vi "STM上位机-Client.vi"() -> ()   [LabVIEW 2015]
uses:
  <vilib>/Math Plots/3D Math Plots/3D Surface/3D Surface XCtrl/3D Surface.xctl
  <vilib>/NI/STM/TCP/TCP Read Options.ctl
  <vilib>/vision/Image Controls.llb/IMAQ Image.ctl
  <vilib>/Analysis/6fits.llb/Curve Fitting Criteria.ctl
  <vilib>/NI/STM/TCP/Read Meta Data (TCP Ref).vi
  <vilib>/NI/STM/TCP/Get Connection Reference (TCP).vi
  <vilib>/NI/STM/TCP/Read Meta Data (TCP Clst).vi
  <vilib>/NI/STM/TCP/Write Message (TCP).vi
  <vilib>/NI/STM/TCP/Read Message (TCP).vi
  <vilib>/Math Plots/3D Math Plots/3D Surface/3D Surface Datatype/Public/Plot Helper (Vector).vi
  <vilib>/NI/STM/NI STM.lvlib
  <vilib>/Math Plots/3D Math Plots/3D Surface/3D Surface Datatype/3D Surface Datatype.lvclass
  <vilib>/Analysis/NI_AALPro.lvlib
panel:
  in  "树形":string(tree)
  in  "Tab Control 3":T1(tab)
  in  "实验人员":string
  in  "实验地点":string
  in  "激光波长":dbl
  in  "自动前进":bool
  in  "自动后退":bool
  in  "中心点":u16(ring) items=["自动", "自动获取质心", "手动取心"]
  in  "步进距离":u16(ring) items=["1mm", "2mm", "4mm", "8mm"]
  in  "触发":bool
  in  "记录数据":bool
  in  "删除数据":bool
  in  "计算M2因子":bool
  in  "是否加中心线":bool
  in  "是否加椭圆线":bool
  out "周长(mm)":dbl
  out "质心坐标X":dbl
  out "质心坐标Y":dbl
  out "面积(mm2)":dbl
  in  "保存数据":bool
  in  "保存边缘检测图像":bool
  in  "保存3D图像":bool
  in  "保存伪彩色图像":bool
  out "位置              长轴半径         短轴半径":string[][](array[string])
  in  "Tab Control 2":T2(tab)
  out "长轴原曲线":dbl[](graph)
  out "长轴拟合曲线":dbl[](graph)
  out "长轴长度":dbl
  out "短轴M2因子":dbl
  out "长轴M2因子":dbl
  out "长轴束腰位置Z0":dbl
  out "长轴束腰直径":dbl
  out "长轴瑞利长度":dbl
  out "长轴光束发散角":dbl
  out "短轴束腰位置Z0":dbl
  out "短轴束腰直径":dbl
  out "短轴瑞利长度":dbl
  out "短轴光束发散角":dbl
  out "手动取点x":i32
  out "是否手动取点":bool
  out "短轴长度":dbl
  out "位置":dbl
  out "3D":u8[](array[numeric])
  out "短轴半径um":dbl
  out "长轴半径um":dbl
  out "短轴原曲线":dbl[](graph)
  out "短轴拟合曲线":dbl[](graph)
  out "纵轴原曲线":dbl[](graph)
  out "纵轴拟合曲线":dbl[](graph)
  out "横轴原曲线":dbl[](graph)
  out "横轴拟合曲线":dbl[](graph)
  in  "Tab Control":enum32{"边缘检测", "3D图像", "伪彩色图像", "三维成像"}(tab)
  out "边缘检测":T3(plugin-control)
  out "3D图像":T3(plugin-control)
  out "伪彩色图像":T3(plugin-control)
  out "三维图像":refnum<class "3D Plot Datatype.lvclass">[](xcontrol) caption="3D Surface"
  in  "读取3D数据":bool
  in  "关闭程序":bool
  out "手动取点y":i32
  # "长轴原曲线"
  # "长轴拟合曲线"
  # "短轴原曲线"
  # "短轴拟合曲线"
  # "纵轴原曲线"
  # "纵轴拟合曲线"
  # "横轴原曲线"
  # "横轴拟合曲线"
  # "三维成像"
  # "-10.00\n\n\n\n-5.00\n\n\n\n-0.00"
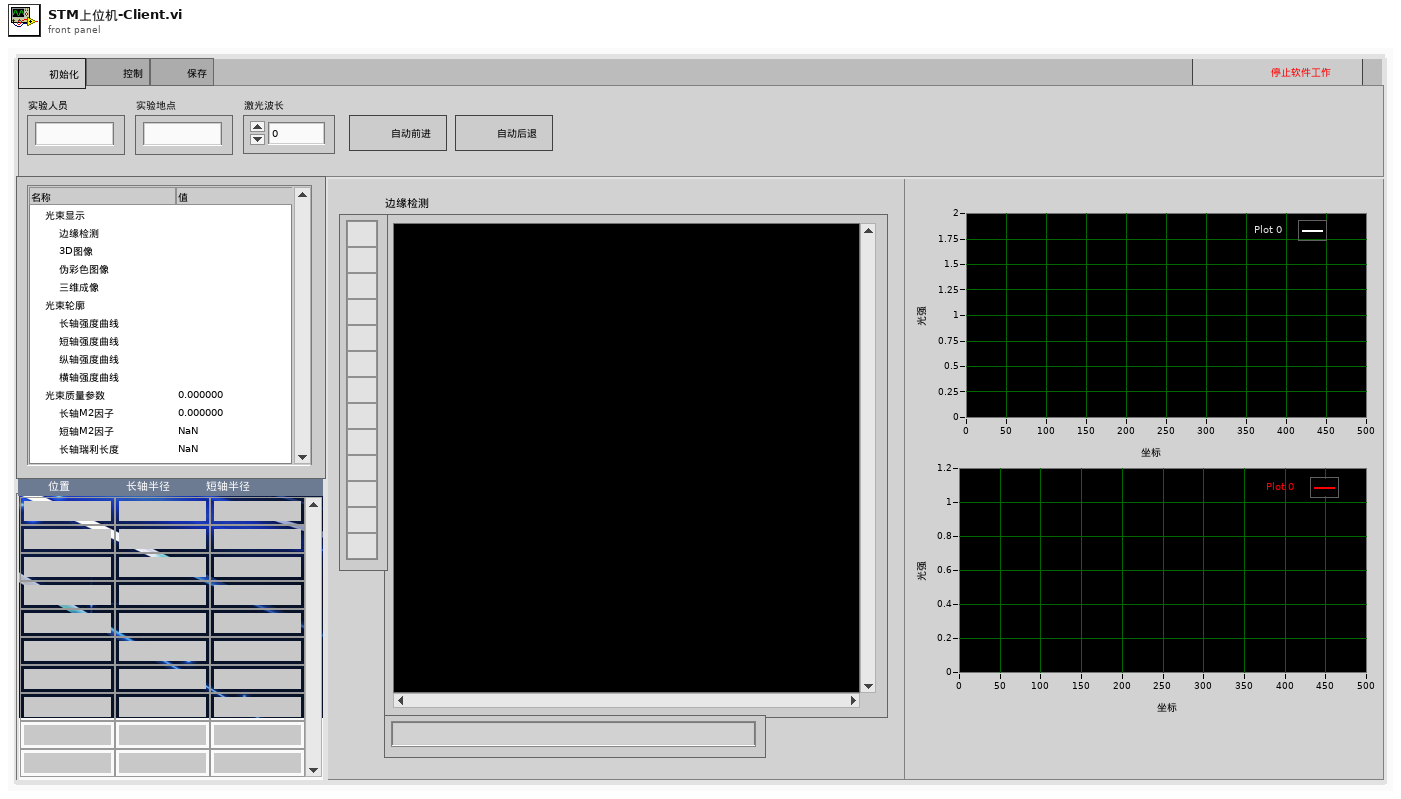
[diagram p1: front panel]
types:
  T1 = enum32{"        初始化", "          控制", "          保存"}
  T2 = enum32{"长轴原曲线", "长轴拟合曲线 ", "短轴原曲线", "短轴拟合曲线", "纵轴原曲线  ", "纵轴拟合曲线  ", "横轴原曲线 ", "横轴拟合曲线 "}
  T3 = typedef "IMAQ Image.ctl" = refnum<image>
  T4 = typedef "NI STM.lvlib/TCP Connection Info.ctl" = cluster{"connection ID":refnum<k5>, "meta data":T5[]}
  T5 = typedef "NI STM.lvlib/MetaDataElement.ctl" = string
  T6 = typedef "NI_AALPro.lvlib/Curve Fitting Criteria.ctl" = u16
  T7 = typedef "NI STM.lvlib/TCP Read Options.ctl" = cluster{"ignore timeout error":bool, "timeout ms (1000)":i32}
  T8 = cluster{"周长":dbl, "面积":dbl, "3D":u8[], "灰度图像":T3, "3D view":T3, "滤波":T3, "边缘检测":T3, "3D图像":T3, "质心坐标X":sgl, "质心坐标Y":sgl, "第一点y值，x=0":dbl, "第二点y值，x=639":dbl, "第一点x值，y=0":dbl, "第二点x值，y=479":dbl, "短轴半径um":dbl, "长轴半径um":dbl, "长轴长度":dbl, "短轴长度":dbl, "短轴原曲线":dbl[], "长轴拟合":dbl[], "纵轴拟合":dbl[], "横轴拟合":dbl[], "长轴原曲线":dbl[], "纵轴原曲线":dbl[], "横轴原曲线":dbl[], "短轴拟合":dbl[], "位置":dbl}
  T9 = cluster{"Global Rectangle":i32[], "Contours":cluster{"Contour Type":u32, "ROI Type":u32, "Points":i32[]}[]}
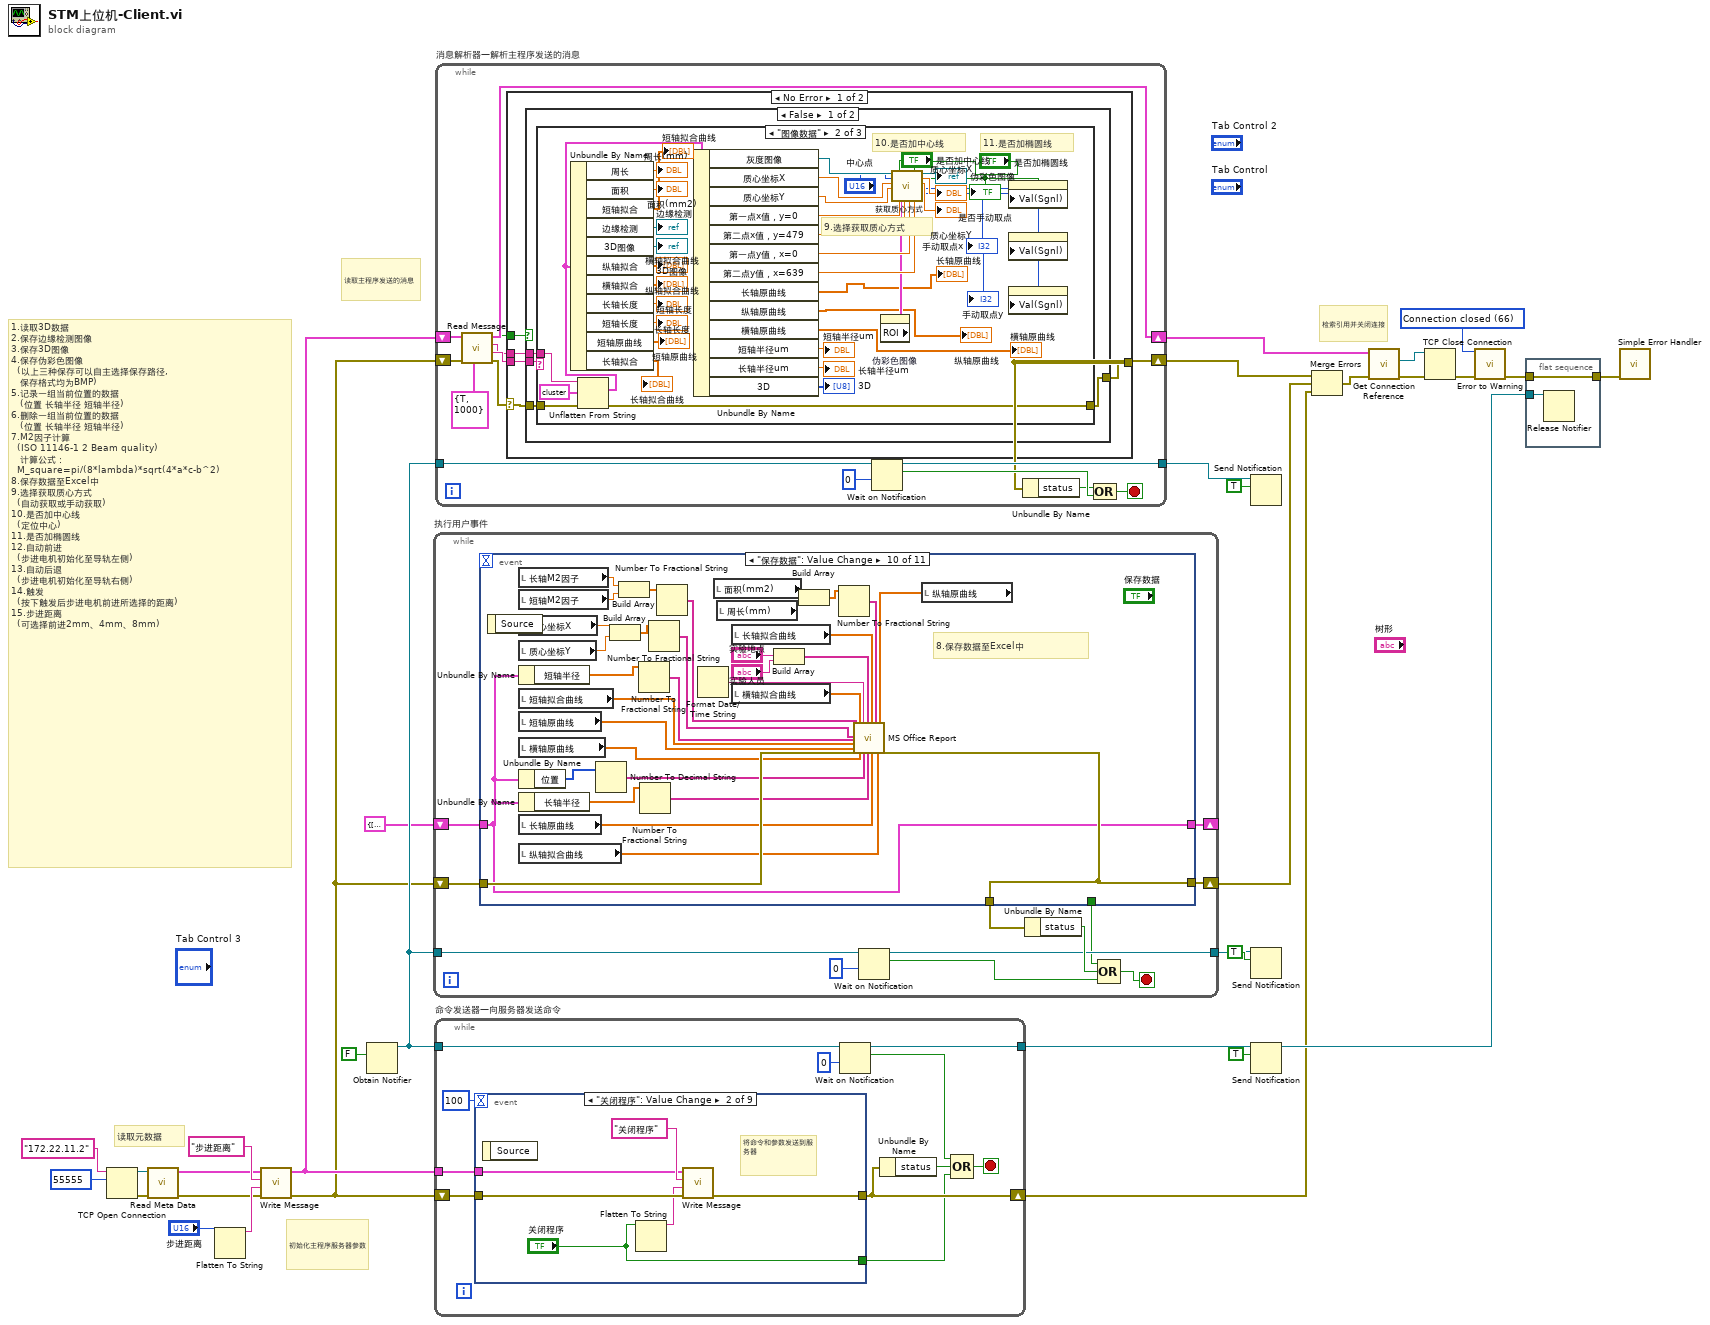
[diagram p0: block diagram]
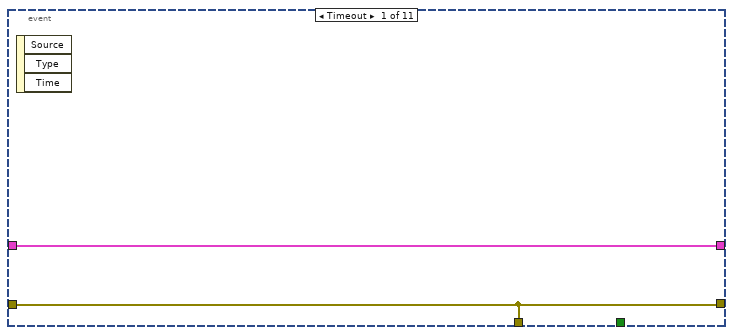
[diagram p2: hidden frame]
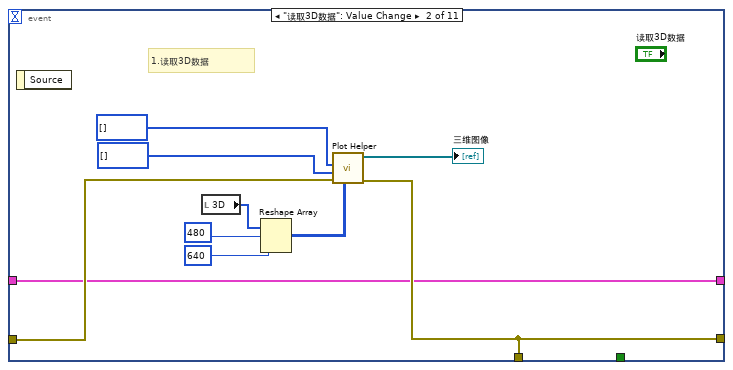
[diagram p3: hidden frame]
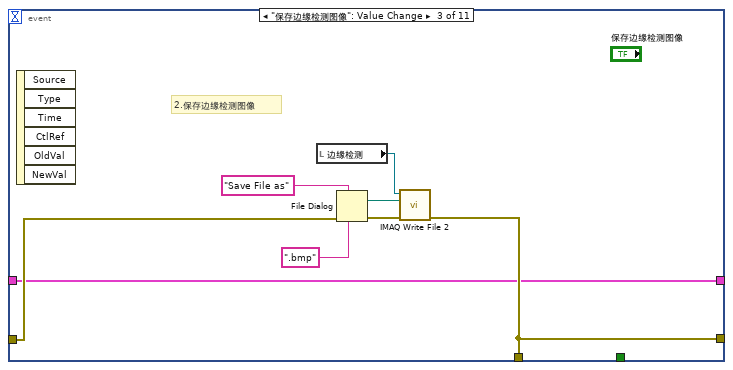
[diagram p4: hidden frame]
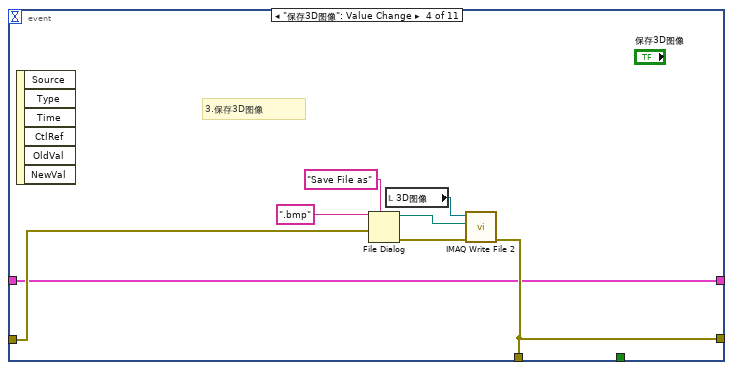
[diagram p5: hidden frame]
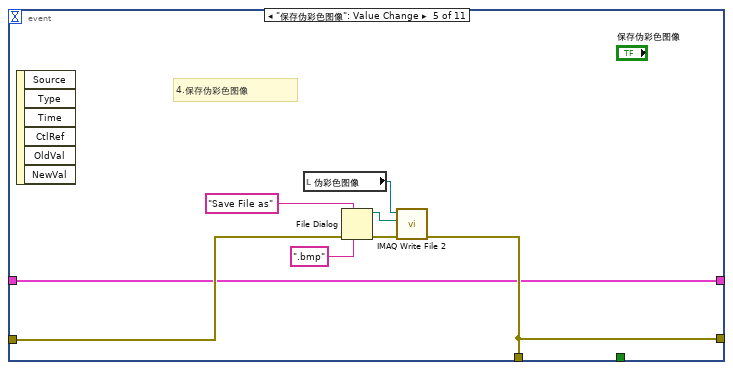
[diagram p6: hidden frame]
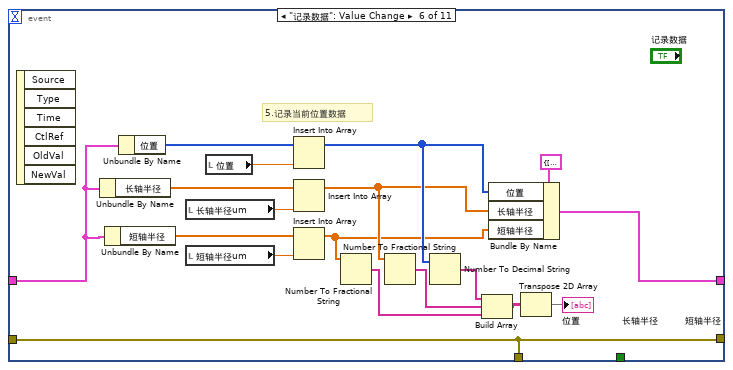
[diagram p7: hidden frame]
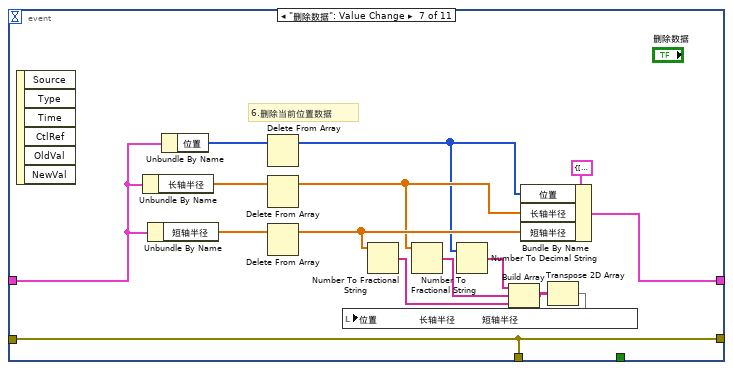
[diagram p8: hidden frame]
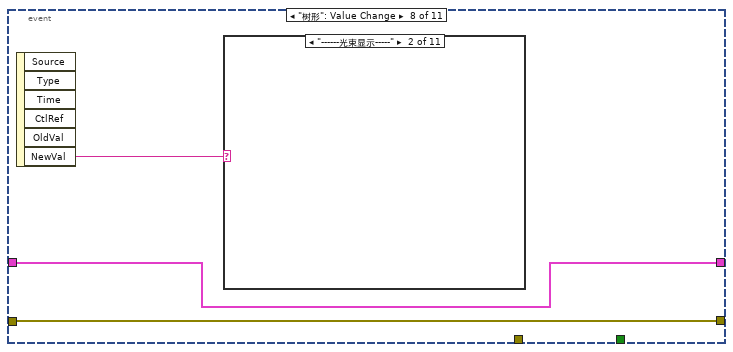
[diagram p9: hidden frame]
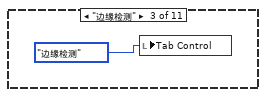
[diagram p11: hidden frame]
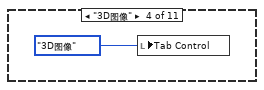
[diagram p12: hidden frame]
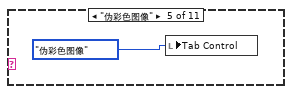
[diagram p13: hidden frame]
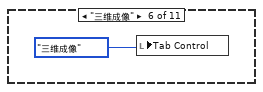
[diagram p14: hidden frame]
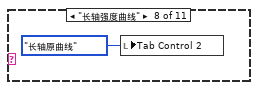
[diagram p16: hidden frame]
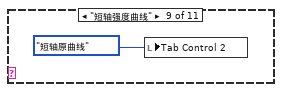
[diagram p17: hidden frame]
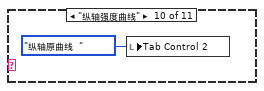
[diagram p18: hidden frame]
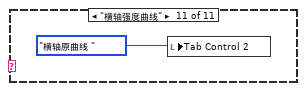
[diagram p19: hidden frame]
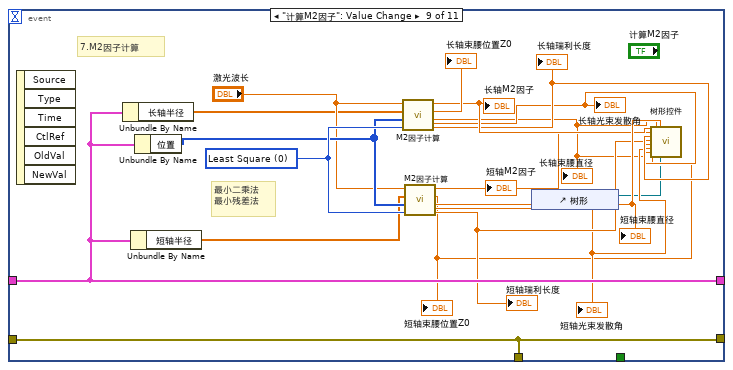
[diagram p20: hidden frame]
diagram:
  w28 = 66 items=["No Error", "Argument Error", "Memory Full", "Out of Zone", "End of File", "File Already Open", "Generic File IO Error", "File Not Found", "File Permission Error", "Disk Full", "Duplicate Path", "Too Many Files Open", "Not Enabled", "Resource File Not Found", "Cannot Add Resource", "Resource Not Found", "Image Not Found", "Image Memory Error", "Pen Does Not Exist", "Config Bad Type", "Config Token Not Found", "Config Parse Error", "Config Memory Error", "Bad External Code Format", "Bad External Code Offset", "External Code Not Present", "Null Window", "Destroy Window Mixup", "Null Menu", "Print Aborted", "Bad Print Record", "Print Driver Error", "Windows Error During Print", "Memory Error During Print", "Print Dialog Error", "Generic Print Error", "Invalid Device Refnum", "Device Not Found", "Device Parameter Error", "Device Unit Error", "Can't Open Device", "Device Call Aborted", "Generic Error", "Cancelled By User", "Object ID Too Low", "Object ID Too High", "Object Not In Heap", "Unknown Heap", "Bad DefProc ID", "DefProc Not In Table", "Message Out Of Range", "Null Method", "Unknown Message", "Manager Call Not Supported", "Bad address", "Connection In progress", "Connection timed out", "Connection is already in progress", "Network attribute not supported", "Network error", "Address in use", "System out of memory", "Connection aborted", "Connection refused", "Connection is not connected", "Connection is already connected", "Connection closed", "Initialize error (interapplication manager)", "Bad occurrence", "Wait on unbound occurrence handler", "Occurrence queue overflow", "Bad path", "Semaphore not signaled", "Unrecognized type (interapplication manager)"] ("1st Error to Convert")
  # "检索引用并关闭连接"
  # "读取元数据"
  # "读取主程序发送的消息"
  # "初始化主程序服务器参数"
  # "1.读取3D数据\n2.保存边缘检测图像\n3.保存3D图像\n4.保存伪彩色图像\n  (以上三种保存可以自主选择保存路径,   \n   保存格式均为BMP)\n5.记录一组当前位置的数据\n   (位置 长轴半径 短轴半径)\n6.删除一组当前位置的数据\n   (位置 长轴半径 短轴半径)\n7.M2因子计算\n  (ISO 11146-1 2 Beam quality)\n   计算公式：\n  M_square=pi/(8*lambda)*sqrt(4*a*c-b^2)\n8.保存数据至Excel中\n9.选择获取质心方式\n  (自动获取或手动获取)\n10.是否加中心线\n  (定位中心)\n11.是否加椭圆线\n12.自动前进\n  (步进电机初始化至导轨左侧)\n13.自动后退\n  (步进电机初始化至导轨右侧)\n14.触发\n  (按下触发后步进电机前进所选择的距离)\n15.步进距离\n  (可选择前进2mm、4mm、8mm)"
  n1 = TCP Open Connection(address="172.22.11.2" ("Target IP Address"), remote port or service name=u16 55555 ("remote port")) -> (connection ID=w32:refnum<k5>, error out=w31:errorcluster)  [unwired: 1 in, 2 out]
  n2 = call-poly "Read Meta Data.vi"("error in"=w31, "connection ID"=w32) -> ("error out"=w3:errorcluster, "connection info out"=w5:T4)  [unwired: 1 in, 7 out]
  n3 = Flatten To String(anything="步进距离") -> (data string=w7:string)  [unwired: 2 in, 3 out]
  n4 = call-poly "Write Message.vi"("error in"=w3, "data"=w7, "name"="步进距离" ("Name"), "connection info in"=w5) -> ("error out"=w2:errorcluster, "connection info out"=w4:T4)  [unwired: 1 in, 5 out]
  n5 = Obtain Notifier(notification data type=FALSE) -> (notifier out=w12:refnum<notifier>)  [unwired: 3 in, 2 out]
  n6 = while "执行用户事件" {
    shift-right: [w36] -> w9
    shift-left: w2 -> [w37]
    tunnel: w12 -> [w42]
    tunnel: [w40] -> w10
    shift-right: [w33] -> _
    shift-left: cluster{"位置":i32[], "长轴半径":dbl[], "短轴半径":dbl[]} {"位置"=[], "长轴半径"=[], "短轴半径"=[]} -> [w38]
    stop <- w39 stop-if-true
    n7 = event shown="[9] \"保存数据\": Value Change" {
      selector: _ -> [_ _ _ _ _ _ _ _ _ _ _]
      dyn-events: _ -> [_ _ _ _ _ _ _ _ _ _ _]
      timeout: _ -> [_ _ _ _ _ _ _ _ _ _ _]
      tunnel: w38 -> [w46 w48 w57 w65 w73 w95 w112 w115 w139 w148 _]
      tunnel: w37 -> [w45 w51 w59 w67 w76 w89 w107 w114 w138 w154 _]
      tunnel: [w45 w49 w58 w66 w75 w89 w107 w114 w138 w153 _] -> w36
      tunnel: [w45 w49 w58 w66 w75 w89 w107 _ w138 w153 _] -> w35
      tunnel: [_ _ _ _ _ _ _ _ _ _ TRUE] -> w34
      tunnel: [w46 w48 w57 w65 w73 w90 w108 w115 w139 w148 _] -> w33
      event Timeout {
        n8 = event-data() -> ()  [unwired: 1 in, 3 out]
      }
      event "读取3D数据": Value Change {
        # "1.读取3D数据"
        n9 = event-data() -> ()  [unwired: 1 in, 1 out]
        n10 = local read "3D"() -> (w50:u8[])
        n11 = Reshape Array(w50, 480 ("dimension size"), 640 ("dimension size")) -> (w54:u8[][])
        n12 = call-poly <vilib>:"Plot Helper.vi"("z matrix"=w54, "error in (no error)"=w51, "y vector"=i32[] [] ("3D"), "x vector"=i32[] [] ("3D")) -> ("error out"=w49:errorcluster, "3D Plot lvclass Array out"=→"三维图像":refnum<class "3D Plot Datatype.lvclass">[])  [unwired: 2 in, 4 out]
      }
      event "保存边缘检测图像": Value Change {
        # "2.保存边缘检测图像"
        n13 = event-data() -> ()  [unwired: 1 in, 6 out]
        n14 = local read "边缘检测"() -> (w60:T3)
        n15 = File Dialog(6:".bmp" ("pattern (all files)"), 7:"Save File as" ("prompt"), 8:w59) -> (0:w61:errorcluster, 3:w64:path)  [unwired: 4 in, 2 out]
        n16 = call-poly "IMAQ Write File 2"("error in (no error)"=w61, "File Path"=w64, "Image"=w60) -> ("error out"=w58:errorcluster)  [unwired: 7 in, 1 out]
      }
      event "保存3D图像": Value Change {
        # "3.保存3D图像"
        n17 = event-data() -> ()  [unwired: 1 in, 6 out]
        n18 = File Dialog(6:".bmp" ("pattern (all files)"), 7:"Save File as" ("prompt"), 8:w67) -> (0:w69:errorcluster, 3:w72:path)  [unwired: 4 in, 2 out]
        n19 = local read "3D图像"() -> (w68:T3)
        n20 = call-poly "IMAQ Write File 2"("error in (no error)"=w69, "File Path"=w72, "Image"=w68) -> ("error out"=w66:errorcluster)  [unwired: 7 in, 1 out]
      }
      event "保存伪彩色图像": Value Change {
        # "4.保存伪彩色图像"
        n21 = event-data() -> ()  [unwired: 1 in, 6 out]
        n22 = local read "伪彩色图像"() -> (w74:T3)
        n23 = File Dialog(6:".bmp" ("pattern (all files)"), 7:"Save File as" ("prompt"), 8:w76) -> (0:w77:errorcluster, 3:w80:path)  [unwired: 4 in, 2 out]
        n24 = call-poly "IMAQ Write File 2"("error in (no error)"=w77, "File Path"=w80, "Image"=w74) -> ("error out"=w75:errorcluster)  [unwired: 7 in, 1 out]
      }
      event "记录数据": Value Change {
        # "5.记录当前位置数据"
        n25 = event-data() -> ()  [unwired: 1 in, 6 out]
        n26 = Unbundle By Name(w95) -> ("长轴半径"=w97:dbl[])
        n27 = Unbundle By Name(w95) -> ("短轴半径"=w98:dbl[])
        n28 = Unbundle By Name(w95) -> ("位置"=w96:i32[])
        n29 = local read "长轴半径um"() -> (w93:dbl)
        n30 = local read "短轴半径um"() -> (w92:dbl)
        n31 = local read "位置"() -> (w94:dbl)
        n32 = Insert Into Array(array=w96, new element=w94) -> (w88:i32[])  [unwired: 1 in]
        n33 = Insert Into Array(array=w97, new element=w93) -> (w87:dbl[])  [unwired: 1 in]
        n34 = Insert Into Array(array=w98, new element=w92) -> (w86:dbl[])  [unwired: 1 in]
        n35 = Number To Fractional String(number=w86) -> (F-format string=w83:string[])  [unwired: 3 in]
        n36 = Number To Fractional String(number=w87) -> (F-format string=w82:string[])  [unwired: 3 in]
        n37 = Number To Decimal String(number=w88) -> (decimal integer string=w81:string[])  [unwired: 1 in]
        n38 = Build Array(w81, w82, w83) -> (w85:string[][])
        n39 = Bundle By Name(cluster=cluster{"位置":i32[], "长轴半径":dbl[], "短轴半径":dbl[]} {"位置"=[], "长轴半径"=[], "短轴半径"=[]}, "位置"=w88, "长轴半径"=w87, "短轴半径"=w86) -> (w90:cluster{"位置":i32[], "长轴半径":dbl[], "短轴半径":dbl[]})
        n40 = Transpose 2D Array(2D array=w85) -> (transposed array=→"位置              长轴半径         短轴半径":string[][])
      }
      event "删除数据": Value Change {
        # "6.删除当前位置数据"
        n41 = event-data() -> ()  [unwired: 1 in, 6 out]
        n42 = Unbundle By Name(w112) -> ("长轴半径"=w110:dbl[])
        n43 = Unbundle By Name(w112) -> ("短轴半径"=w109:dbl[])
        n44 = Unbundle By Name(w112) -> ("位置"=w111:i32[])
        n45 = Delete From Array(array=w111) -> (array with subset deleted=w100:i32[])  [unwired: 2 in, 1 out]
        n46 = Delete From Array(array=w110) -> (array with subset deleted=w101:dbl[])  [unwired: 2 in, 1 out]
        n47 = Delete From Array(array=w109) -> (array with subset deleted=w102:dbl[])  [unwired: 2 in, 1 out]
        n48 = Number To Fractional String(number=w102) -> (F-format string=w105:string[])  [unwired: 3 in]
        n49 = Number To Fractional String(number=w101) -> (F-format string=w104:string[])  [unwired: 3 in]
        n50 = Number To Decimal String(number=w100) -> (decimal integer string=w103:string[])  [unwired: 1 in]
        n51 = Build Array(w103, w104, w105) -> (w106:string[][])
        n52 = Bundle By Name(cluster=cluster{"位置":i32[], "长轴半径":dbl[], "短轴半径":dbl[]} {"位置"=[], "长轴半径"=[], "短轴半径"=[]}, "位置"=w100, "长轴半径"=w101, "短轴半径"=w102) -> (w108:cluster{"位置":i32[], "长轴半径":dbl[], "短轴半径":dbl[]})
        n53 = Transpose 2D Array(2D array=w106) -> (transposed array=w99:string[][])
        n54 = local write "位置              长轴半径         短轴半径"(w99) -> ()
      }
      event "树形": Value Change {
        n55 = event-data() -> ("NewVal"=w116:string)  [unwired: 1 in, 5 out]
        n56 = case shown="\"------光束显示-----\"" w116 {
          frame "假", Default {
          }
          frame "------光束显示-----" {
          }
          frame "边缘检测" {
            n57 = local write "Tab Control"(enum32{"边缘检测", "3D图像", "伪彩色图像", "三维成像"}."边缘检测" ("Tab Control")) -> ()
          }
          frame "3D图像" {
            n58 = local write "Tab Control"(enum32{"边缘检测", "3D图像", "伪彩色图像", "三维成像"}."3D图像" ("Tab Control")) -> ()
          }
          frame "伪彩色图像" {
            n59 = local write "Tab Control"(enum32{"边缘检测", "3D图像", "伪彩色图像", "三维成像"}."伪彩色图像" ("Tab Control")) -> ()
          }
          frame "三维成像" {
            n60 = local write "Tab Control"(enum32{"边缘检测", "3D图像", "伪彩色图像", "三维成像"}."三维成像" ("Tab Control")) -> ()
          }
          frame "------光束轮廓-----" {
          }
          frame "长轴强度曲线" {
            n61 = local write "Tab Control 2"(T2."长轴原曲线" ("Tab Control 2")) -> ()
          }
          frame "短轴强度曲线" {
            n62 = local write "Tab Control 2"(T2."短轴原曲线" ("Tab Control 2")) -> ()
          }
          frame "纵轴强度曲线" {
            n63 = local write "Tab Control 2"(T2."纵轴原曲线  " ("Tab Control 2")) -> ()
          }
          frame "横轴强度曲线" {
            n64 = local write "Tab Control 2"(T2."横轴原曲线 " ("Tab Control 2")) -> ()
          }
        }
      }
      event "计算M2因子": Value Change {
        w142 = T6 0 items=["Least Square", "Least Absolute Residual", "Bisquare"] ("method")
        # "7.M2因子计算"
        # "最小二乘法\n最小残差法"
        n65 = event-data() -> ()  [unwired: 1 in, 6 out]
        n66 = Unbundle By Name(w139) -> ("长轴半径"=w136:dbl[])
        n67 = Unbundle By Name(w139) -> ("短轴半径"=w137:dbl[])
        n68 = Unbundle By Name(w139) -> ("位置"=w141:i32[])
        n69 = call "M2因子计算.vi"("method"=w142, "位置"=w141, "光斑半径"=w136, "激光波长"="激光波长") -> ("瑞利长度"=w131:dbl, "束腰直径"=w127:dbl, "束腰位置Z0"=→"长轴束腰位置Z0":dbl, "M2因子"=w133:dbl, "光束发散角"=w129:dbl)  [unwired: 3 in]
        "长轴M2因子" <- w133
        "长轴束腰直径" <- w127
        "长轴瑞利长度" <- w131
        "长轴光束发散角" <- w129
        n70 = call "M2因子计算.vi"("method"=w142, "位置"=w141, "光斑半径"=w137, "激光波长"="激光波长") -> ("瑞利长度"=w130:dbl, "束腰直径"=w134:dbl, "束腰位置Z0"=w126:dbl, "M2因子"=w132:dbl, "光束发散角"=w128:dbl)  [unwired: 3 in]
        "短轴M2因子" <- w132
        "短轴束腰位置Z0" <- w126
        "短轴束腰直径" <- w134
        "短轴瑞利长度" <- w130
        "短轴光束发散角" <- w128
        n71 = control-ref of="树形"() -> (w125:refnum<vi>)
        n72 = call "树形控件.vi"("长轴M2因子"=w133, "短轴M2因子"=w132, "长轴瑞利长度"=w131, "短轴瑞利长度"=w130, "长轴光束发散角"=w129, "短轴光束发散角"=w128, "长轴束腰位置Z0"=w127, "短轴束腰位置Z0"=w126, "长轴束腰直径"=w127, "短轴束腰直径"=w134, "Tree引用句柄"=w125) -> ()  [unwired: 17 in]
      }
      event "保存数据": Value Change {
        # "8.保存数据至Excel中"
        n73 = event-data() -> ()  [unwired: 1 in, 1 out]
        n74 = local read "长轴M2因子"() -> (w163:dbl)
        n75 = local read "短轴M2因子"() -> (w162:dbl)
        n76 = local read "质心坐标X"() -> (w159:dbl)
        n77 = local read "质心坐标Y"() -> (w158:dbl)
        n78 = Unbundle By Name(w148) -> ("短轴半径"=w151:dbl[])
        n79 = local read "短轴拟合曲线"() -> (w156:dbl[])
        n80 = local read "短轴原曲线"() -> (w155:dbl[])
        n81 = local read "横轴原曲线"() -> (w152:dbl[])
        n82 = Unbundle By Name(w148) -> ("位置"=w147:i32[])
        n83 = Unbundle By Name(w148) -> ("长轴半径"=w146:dbl[])
        n84 = local read "长轴原曲线"() -> (w150:dbl[])
        n85 = local read "纵轴拟合曲线"() -> (w149:dbl[])
        n86 = Number To Decimal String(number=w147) -> (decimal integer string=w145:string[])  [unwired: 1 in]
        n87 = Build Array(w159, w158) -> (w160:dbl[])
        n88 = Build Array(w163, w162) -> (w164:dbl[])
        n89 = Number To Fractional String(number=w151) -> (F-format string=w143:string[])  [unwired: 3 in]
        n90 = Number To Fractional String(number=w146) -> (F-format string=w144:string[])  [unwired: 3 in]
        n91 = Number To Fractional String(number=w160) -> (F-format string=w157:string[])  [unwired: 3 in]
        n92 = Number To Fractional String(number=w164) -> (F-format string=w161:string[])  [unwired: 3 in]
        n93 = Format Date/Time String() -> (date/time string=w166:string)  [unwired: 3 in]
        n94 = local read "面积(mm2)"() -> (w174:dbl)
        n95 = local read "周长(mm)"() -> (w173:dbl)
        n96 = local read "长轴拟合曲线"() -> (w170:dbl[])
        n97 = local read "横轴拟合曲线"() -> (w165:dbl[])
        n98 = Build Array("实验人员", "实验地点") -> (w167:string[])
        n99 = Build Array(w174, w173) -> (w172:dbl[])
        n100 = Number To Fractional String(number=w172) -> (F-format string=w171:string[])  [unwired: 3 in]
        n101 = local read "纵轴原曲线"() -> (w175:dbl[])
        n102 = call "MS Office Report"("M2因子"=w161, "XY"=w157, "短轴半径"=w143, "短轴拟合曲线"=w156, "短轴原曲线"=w155, "error in (no error)"=w154, "横轴拟合曲线"=w165, "横轴原曲线"=w152, "时间"=w166, "位置"=w145, "信息"=w167, "长轴半径"=w144, "长轴拟合曲线"=w170, "长轴原曲线"=w150, "周长与面积"=w171, "纵轴拟合曲线"=w149, "纵轴原曲线"=w175) -> ("error out"=w153:errorcluster)  [unwired: 10 in]
      }
      event "关闭程序": Value Change {
        n103 = event-data() -> ()  [unwired: 1 in, 6 out]
      }
    }
    n104 = Wait on Notification(notifier=w42, timeout in ms (-1)=0) -> (notifier out=w40:refnum<notifier>, notification=w41:bool)  [unwired: 2 in, 2 out]
    n105 = Unbundle By Name(w35) -> ("status"=w44:bool)
    n106 = Compound Arithmetic op=OR(w34, w44, w41) -> (w39:bool)
  }
  n107 = while "命令发送器—向服务器发送命令" {
    tunnel: w4 -> [w187]
    shift-right: [w182] -> w13
    shift-left: w2 -> [w186]
    tunnel: w12 -> [w183]
    tunnel: [w177] -> w17
    stop <- w179 stop-if-true
    n108 = event shown="[1] \"关闭程序\": Value Change" {
      selector: _ -> [_ _ _ _ _ _ _ _ _]
      dyn-events: _ -> [_ _ _ _ _ _ _ _ _]
      timeout: 100 -> [_ _ _ _ _ _ _ _ _]
      tunnel: w187 -> [_ w193 w198 w204 w210 w214 w222 w228 w234]
      tunnel: w186 -> [w188 w192 w197 w203 w209 w215 w221 w227 w233]
      tunnel: [_ "关闭程序" _ _ _ _ _ _ _] -> w180
      tunnel: [w188 w190 w196 w202 w208 w216 w220 w226 w232] -> w182
      event Timeout {
        n109 = event-data() -> ()  [unwired: 2 out]
      }
      event "关闭程序": Value Change {
        # "将命令和参数发送到服务器"
        n110 = event-data() -> ()  [unwired: 2 out]
        n111 = Flatten To String(anything="关闭程序") -> (data string=w191:string)  [unwired: 2 in, 3 out]
        n112 = call-poly "Write Message.vi"("error in"=w192, "data"=w191, "name"="关闭程序" ("Name"), "connection info in"=w193) -> ("error out"=w190:errorcluster)  [unwired: 1 in, 6 out]
      }
      event "自动前进": Value Change {
        # "将命令和参数发送到服务器"
        # "12.自动前进"
        n113 = event-data() -> ()  [unwired: 2 out]
        n114 = Flatten To String(anything="自动前进") -> (data string=w199:string)  [unwired: 2 in, 3 out]
        n115 = call-poly "Write Message.vi"("error in"=w197, "data"=w199, "name"="自动前进" ("Name"), "connection info in"=w198) -> ("error out"=w196:errorcluster)  [unwired: 1 in, 6 out]
      }
      event "自动后退": Value Change {
        # "将命令和参数发送到服务器"
        # "13.自动后退"
        n116 = event-data() -> ()  [unwired: 2 out]
        n117 = Flatten To String(anything="自动后退") -> (data string=w205:string)  [unwired: 2 in, 3 out]
        n118 = call-poly "Write Message.vi"("error in"=w203, "data"=w205, "name"="自动后退" ("Name"), "connection info in"=w204) -> ("error out"=w202:errorcluster)  [unwired: 1 in, 6 out]
      }
      event "触发": Value Change {
        # "将命令和参数发送到服务器"
        # "14.触发"
        n119 = event-data() -> ()  [unwired: 2 out]
        n120 = Flatten To String(anything="触发") -> (data string=w211:string)  [unwired: 2 in, 3 out]
        n121 = call-poly "Write Message.vi"("error in"=w209, "data"=w211, "name"="触发" ("Name"), "connection info in"=w210) -> ("error out"=w208:errorcluster)  [unwired: 1 in, 6 out]
      }
      event "是否手动取点": Value Change {
        # "将命令和参数发送到服务器"
        n122 = event-data() -> ("NewVal"=w213:bool)  [unwired: 1 out]
        n123 = Flatten To String(anything=w213) -> (data string=w217:string)  [unwired: 2 in, 3 out]
        n124 = call-poly "Write Message.vi"("error in"=w215, "data"=w217, "name"="是否手动取点" ("Name"), "connection info in"=w214) -> ("error out"=w216:errorcluster)  [unwired: 1 in, 6 out]
      }
      event "手动取点x": Value Change {
        # "将命令和参数发送到服务器"
        n125 = event-data() -> ("NewVal"=w219:i32)  [unwired: 1 out]
        n126 = Flatten To String(anything=w219) -> (data string=w223:string)  [unwired: 2 in, 3 out]
        n127 = call-poly "Write Message.vi"("error in"=w221, "data"=w223, "name"="手动取点x" ("Name"), "connection info in"=w222) -> ("error out"=w220:errorcluster)  [unwired: 1 in, 6 out]
      }
      event "手动取点y": Value Change {
        # "将命令和参数发送到服务器"
        n128 = event-data() -> ("NewVal"=w225:i32)  [unwired: 1 out]
        n129 = Flatten To String(anything=w225) -> (data string=w229:string)  [unwired: 2 in, 3 out]
        n130 = call-poly "Write Message.vi"("error in"=w227, "data"=w229, "name"="手动取点y" ("Name"), "connection info in"=w228) -> ("error out"=w226:errorcluster)  [unwired: 1 in, 6 out]
      }
      event "步进距离": Value Change {
        # "将命令和参数发送到主程序"
        # "15.步进距离"
        n131 = event-data() -> ("NewVal"=w231:u16)  [unwired: 1 out]
        n132 = Flatten To String(anything=w231) -> (data string=w235:string)  [unwired: 2 in, 3 out]
        n133 = call-poly "Write Message.vi"("error in"=w233, "data"=w235, "name"="步进距离" ("Name"), "connection info in"=w234) -> ("error out"=w232:errorcluster)  [unwired: 1 in, 6 out]
      }
    }
    n134 = Wait on Notification(notifier=w183, timeout in ms (-1)=0) -> (notifier out=w177:refnum<notifier>, notification=w178:bool)  [unwired: 2 in, 2 out]
    n135 = Unbundle By Name(w182) -> ("status"=w181:bool)
    n136 = Compound Arithmetic op=OR(w178, w181, w180) -> (w179:bool)
  }
  n137 = while "消息解析器—解析主程序发送的消息" {
    shift-right: [w249] -> w27
    shift-left: w4 -> [w251]
    shift-right: [w237] -> w24
    shift-left: w2 -> [w250]
    tunnel: w12 -> [w242]
    tunnel: [w240] -> w19
    stop <- w239 stop-if-true
    n138 = call-poly <vilib>:"Read Message.vi"("options"=T7 {"ignore timeout error"=TRUE, "timeout ms (1000)"=1000} ("Options"), "error in"=w250, "connection info in"=w251) -> ("error out"=w245:errorcluster, "name"=w248:T5, "data string"=w247:string, "connection info out"=w249:T4, "timed out?"=w246:bool)  [unwired: 2 in, 2 out]
    n139 = case shown="No Error" w245 {
      selector: w245 -> [w253 w308]
      tunnel: w248 -> [w256 _]
      tunnel: w247 -> [w255 _]
      tunnel: w246 -> [w254 _]
      tunnel: [w252 w308] -> w237
      frame No Error {
        n140 = case shown="False" w254 {
          tunnel: w256 -> [w257 _]
          tunnel: w255 -> [w260 _]
          tunnel: w253 -> [w259 w307]
          tunnel: [w258 w307] -> w252
          frame False {
            n141 = case shown="\"图像数据\"" w257 {
              tunnel: w260 -> [_ w300 w306]
              tunnel: w259 -> [w261 w299 w304]
              tunnel: [w261 w298 w303] -> w258
              frame Default {
              }
              frame "图像数据" {
                # "11.是否加椭圆线"
                # "10.是否加中心线"
                # "9.选择获取质心方式"
                n142 = Unflatten From String(type=T8 {"周长"=0.0, "面积"=0.0, "3D"=[], "灰度图像"=refnum, "3D view"=refnum, "滤波"=refnum, "边缘检测"=refnum, "3D图像"=refnum, "质心坐标X"=0.0, "质心坐标Y"=0.0, "第一点y值，x=0"=0.0, "第二点y值，x=639"=0.0, "第一点x值，y=0"=0.0, "第二点x值，y=479"=0.0, "短轴半径um"=0.0, "长轴半径um"=0.0, "长轴长度"=0.0, "短轴长度"=0.0, "短轴原曲线"=[], "长轴拟合"=[], "纵轴拟合"=[], "横轴拟合"=[], "长轴原曲线"=[], "纵轴原曲线"=[], "横轴原曲线"=[], "短轴拟合"=[], "位置"=0.0}, binary string=w300, error in (no error)=w299) -> (value=w290:T8, error out=w298:errorcluster)  [unwired: 3 out]
                n143 = Unbundle By Name(w290) -> ("周长"=→"周长(mm)":dbl, "面积"=→"面积(mm2)":dbl, "短轴拟合"=→"短轴拟合曲线":dbl[], "边缘检测"=→"边缘检测":T3, "3D图像"=→"3D图像":T3, "纵轴拟合"=→"纵轴拟合曲线":dbl[], "横轴拟合"=→"横轴拟合曲线":dbl[], "长轴长度"=→"长轴长度":dbl, "短轴长度"=→"短轴长度":dbl, "短轴原曲线"=→"短轴原曲线":dbl[], "长轴拟合"=→"长轴拟合曲线":dbl[])
                n144 = Unbundle By Name(w290) -> ("灰度图像"=w286:T3, "质心坐标X"=w283:sgl, "质心坐标Y"=w282:sgl, "第一点x值，y=0"=w281:dbl, "第二点x值，y=479"=w280:dbl, "第一点y值，x=0"=w279:dbl, "第二点y值，x=639"=w278:dbl, "长轴原曲线"=→"长轴原曲线":dbl[], "纵轴原曲线"=→"纵轴原曲线":dbl[], "横轴原曲线"=→"横轴原曲线":dbl[], "短轴半径um"=→"短轴半径um":dbl, "长轴半径um"=→"长轴半径um":dbl, "3D"=→"3D":u8[])
                n145 = property on="伪彩色图像" class="ImageControl"() -> ("ROI"=w274:T9)  [unwired: 2 in, 2 out]
                n146 = call "获取质心方式.vi"("Image"=w286, "中心点"="中心点", "X Centroid"=w283, "Y Centroid"=w282, "ROI"=w274, "是否加中心线"="是否加中心线", "第一点x值，y=0"=w281, "第二点x值,y=479"=w280, "第一点y值，x=0"=w279, "是否加椭圆线"="是否加椭圆线", "第二点y值，x=639"=w278) -> ("是否手动取点"=w273:bool, "Image Out 2"=→"伪彩色图像":T3, "质心坐标X"=→"质心坐标X":dbl, "质心坐标Y"=→"质心坐标Y":dbl, "手动取点x"=w272:i32, "手动取点y"=w271:i32)  [unwired: 2 in, 1 out]
                "手动取点x" <- w272
                "手动取点y" <- w271
                "是否手动取点" <- w273
                n147 = property on="是否手动取点" class="Bool (strict)"("Val(Sgnl)"=w273) -> ()  [unwired: 2 in, 2 out]
                n148 = property on="手动取点x" class="DigNum (strict)"("Val(Sgnl)"=w272) -> ()  [unwired: 2 in, 2 out]
                n149 = property on="手动取点y" class="DigNum (strict)"("Val(Sgnl)"=w271) -> ()  [unwired: 2 in, 2 out]
              }
              frame "步进距离" {
                n150 = Unflatten From String(type=cluster{dbl} {0.0}, binary string=w306, error in (no error)=w304) -> (value=w302:cluster{dbl}, error out=w303:errorcluster)  [unwired: 3 out]
                n151 = Unbundle(w302) -> (→"位置":dbl)
              }
            }
          }
          frame True {
          }
        }
      }
      frame Error {
      }
    }
    n152 = Wait on Notification(notifier=w242, timeout in ms (-1)=0) -> (notifier out=w240:refnum<notifier>, notification=w241:bool)  [unwired: 2 in, 2 out]
    n153 = Unbundle By Name(w237) -> ("status"=w238:bool)
    n154 = Compound Arithmetic op=OR(w238, w241) -> (w239:bool)
  }
  n155 = Send Notification(notification=TRUE, notifier=w19) -> ()  [unwired: 1 in, 2 out]
  n156 = Send Notification(notification=TRUE, notifier=w10) -> ()  [unwired: 1 in, 2 out]
  n157 = Send Notification(notification=TRUE, notifier=w17) -> (notifier out=w14:refnum<notifier>)  [unwired: 1 in, 1 out]
  n158 = Merge Errors(w24, w9, w13) -> (w23:errorcluster)
  n159 = call-poly <vilib>:"Get Connection Reference.vi"("error in"=w23, "connection info in"=w27) -> ("error out"=w25:errorcluster, "connection ID out"=w26:refnum<k5>)  [unwired: 8 out]
  n160 = TCP Close Connection(connection ID=w26, error in (no error)=w25) -> (error out=w22:errorcluster)  [unwired: 2 out]
  n161 = call <vilib>:"Error to Warning.vi"("1st Error to Convert"=w28, "error in"=w22) -> ("warning out"=w16:errorcluster)  [unwired: 3 in, 10 out]
  n162 = flat-sequence {
    tunnel: w14 -> [w310]
    tunnel: w16 -> [w309]
    tunnel: [w309] -> w15
    frame #0 {
      n163 = Release Notifier(notifier=w310) -> ()  [unwired: 2 in, 3 out]
    }
  }
  n164 = call <vilib>:"Simple Error Handler.vi"("error in (no error)"=w15) -> ()  [unwired: 4 in, 5 out]
